vi "DOCK_LOGIN_scan_barcode.vi"(8 "error_in":errorcluster, 11 "all_config_info":T1={"main_ini_file"={"SQL Driver"="", "SQL Server"="", "SQL Database"="", "SQL UID"="", "Reference table"="", "Reference history"="", "Archivisation CFG table"="", "Archivisation CFG history"="", "User table"="", "User history"="", "default language"="", "SCANNER COM port"=0, "SCANNER Baud rate"=0, "SCANNER Data bits"=0, "SCANNER Pairity"=enum."None", "SCANNER Stop bits"=0, "SCANNER Flow control"=0, "SCANNER Termination char"=10, "PRINTER PC port"=0, "PRINTER IP"="", "PRINTER port"=0, "PRINTER Keep alive timer [ms]"=0, "logout timeout [ms]"=0}, "SQL Password"="", "PRINTER Label"="", "PRINTER Template"="", "Last Label"="", "queue_refnums"={"MAIN_queue"=refnum, "SCANNER_queue"=refnum, "SCANNER_login"=refnum, "PRINTER_queue"=refnum}} {"main_ini_file"."SCANNER Flow control" items=["None"=0, "XON/XOFF"=1, "RTS/CTS"=2, "DTR/DSR"=4]; "main_ini_file"."SCANNER Stop bits" items=["1.0"=10, "1.5"=15, "2.0"=20]}) -> (0 "error_out":errorcluster, 2 "Canceled?":bool, 3 "barcode":string)   [LabVIEW 2019]
uses:
  ini/typedef/DOCK_all_config_info.ctl
  ini/typedef/DOCK_main_ini_file.ctl
  queues/typedef/DOCK_queue_refnums.ctl
  queues/typedef/DOCK_MAIN_queue_element.ctl
  DOCK_MAIN_sequence_state.ctl
  queues/typedef/DOCK_SCANNER_queue_element.ctl
  SCANNER/DOCK_SCANNER_sequence_state.ctl
  queues/typedef/DOCK_PRINTER_queue_element.ctl
  PRINTER/DOCK_PRINTER_sequence_state.ctl
  _misc/AULocalize/SubVIs/RegisterVI.vi
panel:
  out "waiting_for_barcode_scan_msg":string caption="Waiting for barcode scan..."
  in  "cancel_barcode_scan":bool
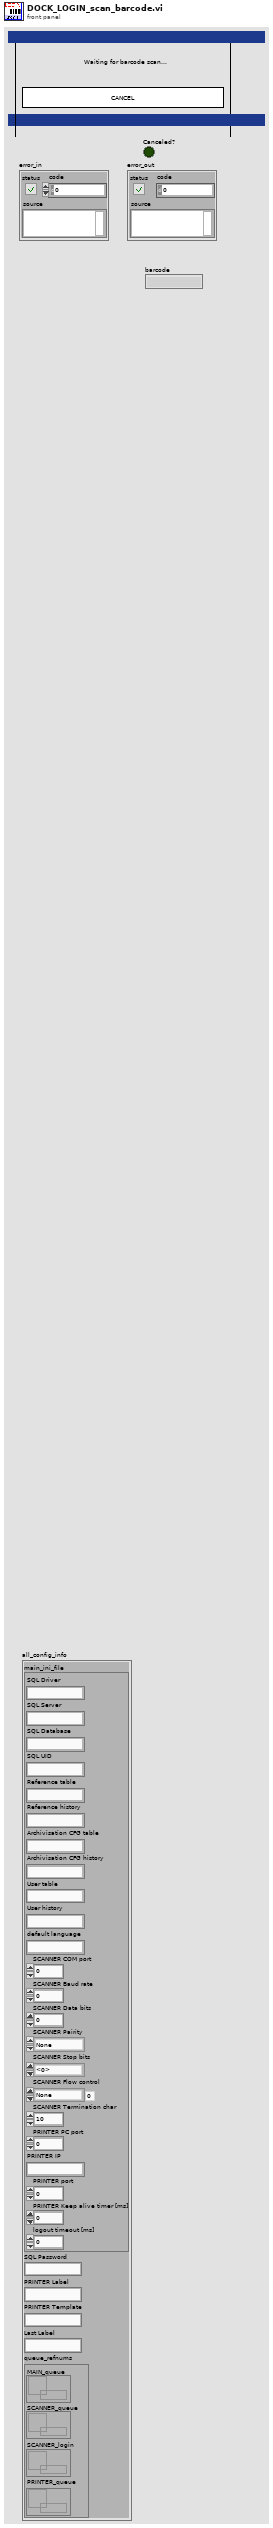
[diagram p1: front panel]
types:
  T1 = typedef "DOCK_all_config_info.ctl" = cluster{"main_ini_file":T2, "SQL Password":string, "PRINTER Label":string, "PRINTER Template":string, "Last Label":string, "queue_refnums":T3}
  T2 = typedef "DOCK_main_ini_file.ctl" = cluster{"SQL Driver":string, "SQL Server":string, "SQL Database":string, "SQL UID":string, "Reference table":string, "Reference history":string, "Archivisation CFG table":string, "Archivisation CFG history":string, "User table":string, "User history":string, "default language":string, "SCANNER COM port":u16, "SCANNER Baud rate":u32, "SCANNER Data bits":u16, "SCANNER Pairity":enum16{"None", "Odd", "Even", "Mark", "Space"}, "SCANNER Stop bits":u16, "SCANNER Flow control":u16, "SCANNER Termination char":u8, "PRINTER PC port":u16, "PRINTER IP":string, "PRINTER port":u16, "PRINTER Keep alive timer [ms]":i32, "logout timeout [ms]":i32}
  T3 = typedef "DOCK_queue_refnums.ctl" = cluster{"MAIN_queue":refnum<queue>, "SCANNER_queue":refnum<queue>, "SCANNER_login":refnum<queue>, "PRINTER_queue":refnum<queue>}
  T4 = typedef "DOCK_SCANNER_queue_element.ctl" = cluster{"state":T5, "variable":variant}
  T5 = typedef "DOCK_SCANNER_sequence_state.ctl" = enum16{"initialize", "get_next_state", "read", "error", "stop"}
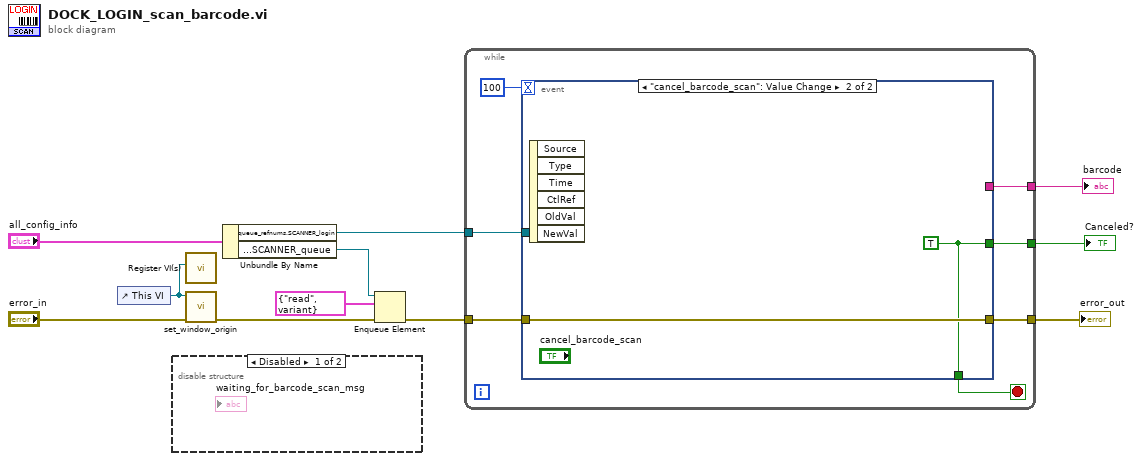
[diagram p0: block diagram]
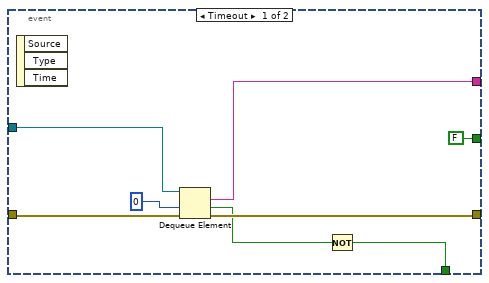
[diagram p3: hidden frame]
diagram:
  n1 = control-ref of="This VI"() -> (w1:refnum<vi>)
  n2 = disable-structure shown="Disabled" {
    frame Disabled {
    }
    frame Enabled {
    }
  }
  n3 = call-poly "Register VI(s).vi"("VI Ref"=w1) -> ()  [unwired: 9 in, 2 out]
  n4 = call "set_window_origin.vi"("error_in"="error_in", "this_vi_reference"=w1) -> ("error_out"=w6:errorcluster)  [unwired: 9 in]
  n5 = Unbundle By Name("all_config_info") -> ("queue_refnums.SCANNER_login"=w8:refnum<queue>, "queue_refnums.SCANNER_queue"=w4:refnum<queue>)
  n6 = Enqueue Element(queue=w4, element=T4 {"state"=enum."read", "variable"=variant}, error in (no error)=w6) -> (error out=w5:errorcluster)  [unwired: 1 in, 2 out]
  n7 = while {
    tunnel: w5 -> [w18]
    tunnel: [w17] -> w11
    tunnel: w8 -> [w14]
    tunnel: [w13] -> w7
    tunnel: [w12] -> w3
    stop <- w15 stop-if-true
    n8 = event shown="[1] \"cancel_barcode_scan\": Value Change" {
      selector: _ -> [_ _]
      dyn-events: _ -> [_ _]
      timeout: 100 -> [_ _]
      tunnel: w18 -> [w25 w28]
      tunnel: [w24 w28] -> w17
      tunnel: [w20 w27] -> w15
      tunnel: w14 -> [w26 _]
      tunnel: [w21 _] -> w13
      tunnel: [FALSE w27] -> w12
      event Timeout {
        n9 = event-data() -> ()  [unwired: 1 in, 3 out]
        n10 = Dequeue Element(queue=w26, timeout in ms (-1)=0, error in (no error)=w25) -> (element=w21:string, timed out?=w22:bool, error out=w24:errorcluster)  [unwired: 1 out]
        n11 = Not(x=w22) -> (.not. x?=w20:bool)
      }
      event "cancel_barcode_scan": Value Change {
        w27 = TRUE
        n12 = event-data() -> ()  [unwired: 1 in, 6 out]
      }
    }
  }
  "error_out" <- w11
  "barcode" <- w7
  "Canceled?" <- w3
